vi "MSEncoder SubVI DynamicTimeout_Add.vi"(8 "error in (no error)":errorcluster, 10 "Timeout_ms":i32, 11 "MSEncoder":refnum<class "MSEncoder.lvclass">) -> (0 "error out":errorcluster, 3 "MSEncoder":refnum<class "MSEncoder.lvclass">)   [LabVIEW 2018, in "MSEncoder.lvclass"]
uses:
  MSEncoder.lvclass
  MSEncoder.lvclass/MSEncoder.ctl
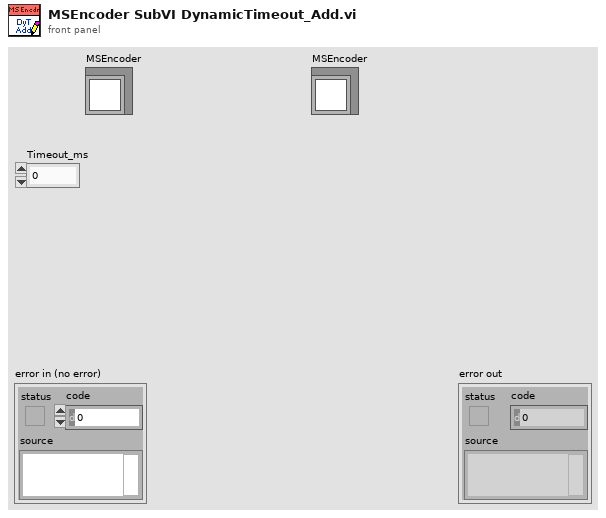
[diagram p1: front panel]
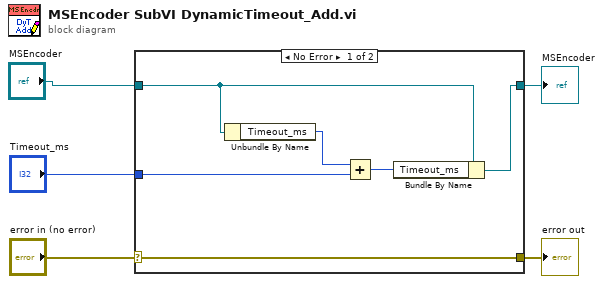
[diagram p0: block diagram]
diagram:
  n1 = case shown="No Error" "error in (no error)" {
    selector: "error in (no error)" -> [w11 w12]
    tunnel: [w11 w12] -> w4
    tunnel: [w10 w13] -> w1
    tunnel: "MSEncoder" -> [w8 w13]
    tunnel: "Timeout_ms" -> [w9 _]
    frame No Error {
      n2 = Unbundle By Name(w8) -> ("Timeout_ms"=w6:i32)
      n3 = Add(x=w6, y=w9) -> (x+y=w7:i32)
      n4 = Bundle By Name(cluster=w8, "Timeout_ms"=w7) -> (w10:refnum<class "MSEncoder.lvclass">)
    }
    frame Error {
    }
  }
  "error out" <- w4
  "MSEncoder" <- w1
